vi "AlliGator Update Menu.vi"(8 "Error In":errorcluster, 11 "Menu in":refnum<k9>) -> (0 "Error Out":errorcluster)   [LabVIEW 2021, in "AlliGator GUI.lvlib"]
doc: "Updates AlliGator menu upon activation, in order to set checkmarks and include dynamic menu items such as Python plugins."
uses:
  AlliGator GUI.lvlib
  Globals, Variables, Constants/AlliGator Globals.vi
  Globals, Variables, Constants/AlliGator Globals, Variables & Constants.lvlib
  Python Plugins API/AlliGator Python Plugins.lvlib
panel:
  # "see the AlliGator License on the block diagram (Ctrl+E or Window:Show Block Diagram)"
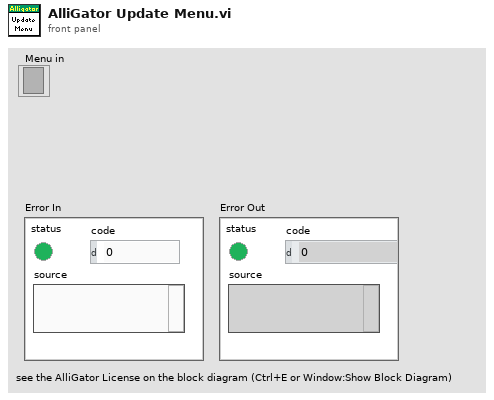
[diagram p1: front panel]
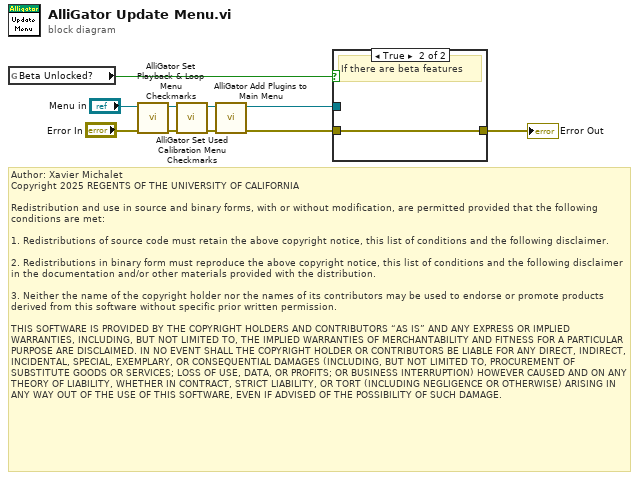
[diagram p0: block diagram]
diagram:
  # "Author: Xavier Michalet\nCopyright 2025 REGENTS OF THE UNIVERSITY OF CALIFORNIA\n\nRedistribution and use in source and binary forms, with or without modification, are permitted provided that the following conditions are met:\n\n1. Redistributions of source code must retain the above copyright notice, this list of conditions and the following disclaimer.\n\n2. Redistributions in binary form must reproduce the above copyright notice, this list of conditions and the following disclaimer in the documentation and/or other materials provided with the distribution.\n\n3. Neither the name of the copyright holder nor the names of its contributors may be used to endorse or promote products derived from this software without specific prior written permission.\n\nTHIS SOFTWARE IS PROVIDED BY THE COPYRIGHT HOLDERS AND CONTRIBUTORS “AS IS” AND ANY EXPRESS OR IMPLIED WARRANTIES, INCLUDING, BUT NOT LIMITED TO, THE IMPLIED WARRANTIES OF MERCHANTABILITY AND FITNESS FOR A PARTICULAR PURPOSE ARE DISCLAIMED. IN NO EVENT SHALL THE COPYRIGHT HOLDER OR CONTRIBUTORS BE LIABLE FOR ANY DIRECT, INDIRECT, INCIDENTAL, SPECIAL, EXEMPLARY, OR CONSEQUENTIAL DAMAGES (INCLUDING, BUT NOT LIMITED TO, PROCUREMENT OF SUBSTITUTE GOODS OR SERVICES; LOSS OF USE, DATA, OR PROFITS; OR BUSINESS INTERRUPTION) HOWEVER CAUSED AND ON ANY THEORY OF LIABILITY, WHETHER IN CONTRACT, STRICT LIABILITY, OR TORT (INCLUDING NEGLIGENCE OR OTHERWISE) ARISING IN ANY WAY OUT OF THE USE OF THIS SOFTWARE, EVEN IF ADVISED OF THE POSSIBILITY OF SUCH DAMAGE."
  n1 = global read "AlliGator Globals.vi" "Beta Unlocked?"() -> (w8:bool)
  n2 = call "AlliGator Set Playback & Loop Menu Checkmarks.vi"("Error In"="Error In", "Menu in"="Menu in") -> ("Error Out"=w3:errorcluster, "Menu out"=w4:refnum<k9>)  [unwired: 8 in]
  n3 = call "AlliGator Set Used Calibration Menu Checkmarks.vi"("Error In"=w3, "Menu in"=w4) -> ("Error Out"=w2:errorcluster, "Menu out"=w1:refnum<k9>)  [unwired: 8 in]
  n4 = call "AlliGator Add Plugins to Main Menu.vi"("error in (no error)"=w2, "Menu in"=w1) -> ("error out"=w7:errorcluster, "Menu out"=w5:refnum<k9>)  [unwired: 8 in]
  n5 = case shown="True" w8 {
    tunnel: w7 -> [w11 w12]
    tunnel: [w11 w12] -> w6
    tunnel: w5 -> [_ _]
    frame False {
    }
    frame True {
      # "If there are beta features"
    }
  }
  "Error Out" <- w6
